vi "Auto Segement Extract.vi"(4 "Save Path":path, 5 "Sensor Data Array":dbl[][](array[numeric]), 7 "Title":string) -> (0 "End":dbl, 1 "Trimmed Segment":dbl[][](graph), 2 "No Peak Located":bool, 3 "Start":dbl)   [LabVIEW 2020]
uses:
  <vilib>/Utility/miscctls.llb/LVCursorListTypeDef.ctl
  <vilib>/Analysis/NI_AAL_SigProc.lvlib
panel:
  in  "OK Button":bool
  out "Last Sensor":dbl[](graph)
  out "First Sensor":dbl[](graph)
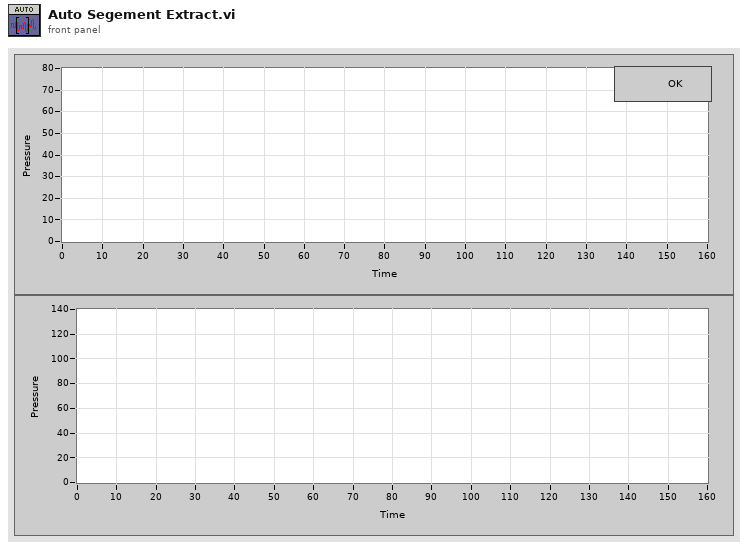
[diagram p1: front panel]
types:
  T1 = enum16{"open", "replace", "create", "open or create", "replace or create", "replace or create with confirmation"}
  T2 = typedef "LVCursorListTypeDef.ctl" = cluster{"Name":string, "Color":u32, "Style":u8, "Point Style":u8, "Name Visible":bool, "Allow Drag":bool, "Cursor Mode":u32, "Plot":i32, "Index":i32, "Position":cluster{"X":dbl, "Y":dbl}, "X Scale":u32, "Y Scale":u32, "Watch Plots":i32[], "Watch All Plots":bool, "Plot Area":i32, "Label Offset":cluster{"X":dbl, "Y":dbl}}[]
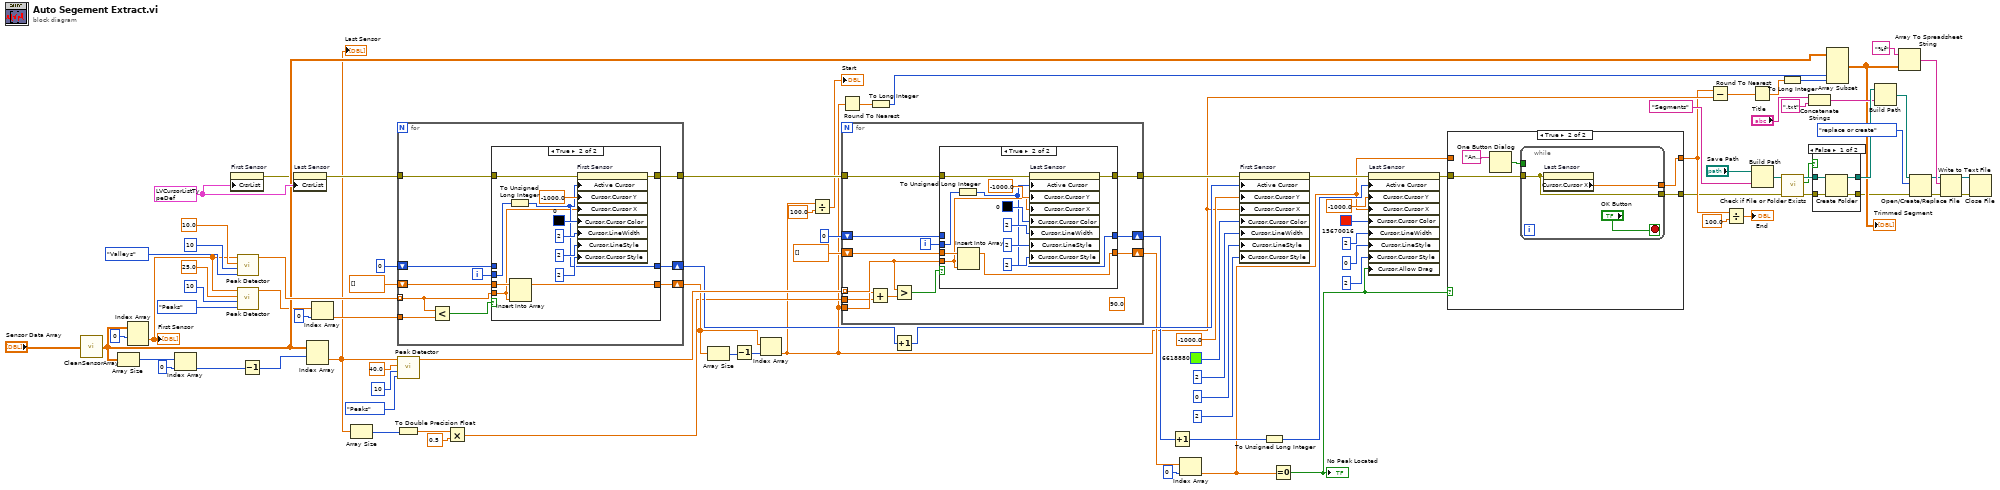
[diagram p0: block diagram]
diagram:
  w83 = T2 [{"Name"="", "Color"=0, "Style"=0, "Point Style"=0, "Name Visible"=FALSE, "Allow Drag"=FALSE, "Cursor Mode"=0, "Plot"=0, "Index"=0, "Position"={"X"=0.0, "Y"=0.0}, "X Scale"=0, "Y Scale"=0, "Watch Plots"=[], "Watch All Plots"=FALSE, "Plot Area"=0, "Label Offset"={"X"=0.0, "Y"=0.0}}, {"Name"="", "Color"=0, "Style"=0, "Point Style"=0, "Name Visible"=FALSE, "Allow Drag"=FALSE, "Cursor Mode"=0, "Plot"=0, "Index"=0, "Position"={"X"=0.0, "Y"=0.0}, "X Scale"=0, "Y Scale"=0, "Watch Plots"=[], "Watch All Plots"=FALSE, "Plot Area"=0, "Label Offset"={"X"=0.0, "Y"=0.0}}, {"Name"="", "Color"=0, "Style"=0, "Point Style"=0, "Name Visible"=FALSE, "Allow Drag"=FALSE, "Cursor Mode"=0, "Plot"=0, "Index"=0, "Position"={"X"=0.0, "Y"=0.0}, "X Scale"=0, "Y Scale"=0, "Watch Plots"=[], "Watch All Plots"=FALSE, "Plot Area"=0, "Label Offset"={"X"=0.0, "Y"=0.0}}, {"Name"="", "Color"=0, "Style"=0, "Point Style"=0, "Name Visible"=FALSE, "Allow Drag"=FALSE, "Cursor Mode"=0, "Plot"=0, "Index"=0, "Position"={"X"=0.0, "Y"=0.0}, "X Scale"=0, "Y Scale"=0, "Watch Plots"=[], "Watch All Plots"=FALSE, "Plot Area"=0, "Label Offset"={"X"=0.0, "Y"=0.0}}, {"Name"="", "Color"=0, "Style"=0, "Point Style"=0, "Name Visible"=FALSE, "Allow Drag"=FALSE, "Cursor Mode"=0, "Plot"=0, "Index"=0, "Position"={"X"=0.0, "Y"=0.0}, "X Scale"=0, "Y Scale"=0, "Watch Plots"=[], "Watch All Plots"=FALSE, "Plot Area"=0, "Label Offset"={"X"=0.0, "Y"=0.0}}, {"Name"="", "Color"=0, "Style"=0, "Point Style"=0, "Name Visible"=FALSE, "Allow Drag"=FALSE, "Cursor Mode"=0, "Plot"=0, "Index"=0, "Position"={"X"=0.0, "Y"=0.0}, "X Scale"=0, "Y Scale"=0, "Watch Plots"=[], "Watch All Plots"=FALSE, "Plot Area"=0, "Label Offset"={"X"=0.0, "Y"=0.0}}, {"Name"="", "Color"=0, "Style"=0, "Point Style"=0, "Name Visible"=FALSE, "Allow Drag"=FALSE, "Cursor Mode"=0, "Plot"=0, "Index"=0, "Position"={"X"=0.0, "Y"=0.0}, "X Scale"=0, "Y Scale"=0, "Watch Plots"=[], "Watch All Plots"=FALSE, "Plot Area"=0, "Label Offset"={"X"=0.0, "Y"=0.0}}, {"Name"="", "Color"=0, "Style"=0, "Point Style"=0, "Name Visible"=FALSE, "Allow Drag"=FALSE, "Cursor Mode"=0, "Plot"=0, "Index"=0, "Position"={"X"=0.0, "Y"=0.0}, "X Scale"=0, "Y Scale"=0, "Watch Plots"=[], "Watch All Plots"=FALSE, "Plot Area"=0, "Label Offset"={"X"=0.0, "Y"=0.0}}, {"Name"="", "Color"=0, "Style"=0, "Point Style"=0, "Name Visible"=FALSE, "Allow Drag"=FALSE, "Cursor Mode"=0, "Plot"=0, "Index"=0, "Position"={"X"=0.0, "Y"=0.0}, "X Scale"=0, "Y Scale"=0, "Watch Plots"=[], "Watch All Plots"=FALSE, "Plot Area"=0, "Label Offset"={"X"=0.0, "Y"=0.0}}, {"Name"="", "Color"=0, "Style"=0, "Point Style"=0, "Name Visible"=FALSE, "Allow Drag"=FALSE, "Cursor Mode"=0, "Plot"=0, "Index"=0, "Position"={"X"=0.0, "Y"=0.0}, "X Scale"=0, "Y Scale"=0, "Watch Plots"=[], "Watch All Plots"=FALSE, "Plot Area"=0, "Label Offset"={"X"=0.0, "Y"=0.0}}, {"Name"="", "Color"=0, "Style"=0, "Point Style"=0, "Name Visible"=FALSE, "Allow Drag"=FALSE, "Cursor Mode"=0, "Plot"=0, "Index"=0, "Position"={"X"=0.0, "Y"=0.0}, "X Scale"=0, "Y Scale"=0, "Watch Plots"=[], "Watch All Plots"=FALSE, "Plot Area"=0, "Label Offset"={"X"=0.0, "Y"=0.0}}, {"Name"="", "Color"=0, "Style"=0, "Point Style"=0, "Name Visible"=FALSE, "Allow Drag"=FALSE, "Cursor Mode"=0, "Plot"=0, "Index"=0, "Position"={"X"=0.0, "Y"=0.0}, "X Scale"=0, "Y Scale"=0, "Watch Plots"=[], "Watch All Plots"=FALSE, "Plot Area"=0, "Label Offset"={"X"=0.0, "Y"=0.0}}, {"Name"="", "Color"=0, "Style"=0, "Point Style"=0, "Name Visible"=FALSE, "Allow Drag"=FALSE, "Cursor Mode"=0, "Plot"=0, "Index"=0, "Position"={"X"=0.0, "Y"=0.0}, "X Scale"=0, "Y Scale"=0, "Watch Plots"=[], "Watch All Plots"=FALSE, "Plot Area"=0, "Label Offset"={"X"=0.0, "Y"=0.0}}, {"Name"="", "Color"=0, "Style"=0, "Point Style"=0, "Name Visible"=FALSE, "Allow Drag"=FALSE, "Cursor Mode"=0, "Plot"=0, "Index"=0, "Position"={"X"=0.0, "Y"=0.0}, "X Scale"=0, "Y Scale"=0, "Watch Plots"=[], "Watch All Plots"=FALSE, "Plot Area"=0, "Label Offset"={"X"=0.0, "Y"=0.0}}, {"Name"="", "Color"=0, "Style"=0, "Point Style"=0, "Name Visible"=FALSE, "Allow Drag"=FALSE, "Cursor Mode"=0, "Plot"=0, "Index"=0, "Position"={"X"=0.0, "Y"=0.0}, "X Scale"=0, "Y Scale"=0, "Watch Plots"=[], "Watch All Plots"=FALSE, "Plot Area"=0, "Label Offset"={"X"=0.0, "Y"=0.0}}, {"Name"="", "Color"=0, "Style"=0, "Point Style"=0, "Name Visible"=FALSE, "Allow Drag"=FALSE, "Cursor Mode"=0, "Plot"=0, "Index"=0, "Position"={"X"=0.0, "Y"=0.0}, "X Scale"=0, "Y Scale"=0, "Watch Plots"=[], "Watch All Plots"=FALSE, "Plot Area"=0, "Label Offset"={"X"=0.0, "Y"=0.0}}, {"Name"="", "Color"=0, "Style"=0, "Point Style"=0, "Name Visible"=FALSE, "Allow Drag"=FALSE, "Cursor Mode"=0, "Plot"=0, "Index"=0, "Position"={"X"=0.0, "Y"=0.0}, "X Scale"=0, "Y Scale"=0, "Watch Plots"=[], "Watch All Plots"=FALSE, "Plot Area"=0, "Label Offset"={"X"=0.0, "Y"=0.0}}, {"Name"="", "Color"=0, "Style"=0, "Point Style"=0, "Name Visible"=FALSE, "Allow Drag"=FALSE, "Cursor Mode"=0, "Plot"=0, "Index"=0, "Position"={"X"=0.0, "Y"=0.0}, "X Scale"=0, "Y Scale"=0, "Watch Plots"=[], "Watch All Plots"=FALSE, "Plot Area"=0, "Label Offset"={"X"=0.0, "Y"=0.0}}, {"Name"="", "Color"=0, "Style"=0, "Point Style"=0, "Name Visible"=FALSE, "Allow Drag"=FALSE, "Cursor Mode"=0, "Plot"=0, "Index"=0, "Position"={"X"=0.0, "Y"=0.0}, "X Scale"=0, "Y Scale"=0, "Watch Plots"=[], "Watch All Plots"=FALSE, "Plot Area"=0, "Label Offset"={"X"=0.0, "Y"=0.0}}, {"Name"="", "Color"=0, "Style"=0, "Point Style"=0, "Name Visible"=FALSE, "Allow Drag"=FALSE, "Cursor Mode"=0, "Plot"=0, "Index"=0, "Position"={"X"=0.0, "Y"=0.0}, "X Scale"=0, "Y Scale"=0, "Watch Plots"=[], "Watch All Plots"=FALSE, "Plot Area"=0, "Label Offset"={"X"=0.0, "Y"=0.0}}, {"Name"="", "Color"=0, "Style"=0, "Point Style"=0, "Name Visible"=FALSE, "Allow Drag"=FALSE, "Cursor Mode"=0, "Plot"=0, "Index"=0, "Position"={"X"=0.0, "Y"=0.0}, "X Scale"=0, "Y Scale"=0, "Watch Plots"=[], "Watch All Plots"=FALSE, "Plot Area"=0, "Label Offset"={"X"=0.0, "Y"=0.0}}, {"Name"="", "Color"=0, "Style"=0, "Point Style"=0, "Name Visible"=FALSE, "Allow Drag"=FALSE, "Cursor Mode"=0, "Plot"=0, "Index"=0, "Position"={"X"=0.0, "Y"=0.0}, "X Scale"=0, "Y Scale"=0, "Watch Plots"=[], "Watch All Plots"=FALSE, "Plot Area"=0, "Label Offset"={"X"=0.0, "Y"=0.0}}, {"Name"="Marker", "Color"=0, "Style"=0, "Point Style"=0, "Name Visible"=FALSE, "Allow Drag"=FALSE, "Cursor Mode"=0, "Plot"=0, "Index"=0, "Position"={"X"=0.0, "Y"=0.0}, "X Scale"=0, "Y Scale"=0, "Watch Plots"=[], "Watch All Plots"=FALSE, "Plot Area"=0, "Label Offset"={"X"=0.0, "Y"=0.0}}] ("Cursor List")
  n1 = call "CleanSensorArray.vi"("Sensor Data Array"="Sensor Data Array") -> ("Clean Array"=w77:dbl[][])  [unwired: 4 in]
  n2 = Array Size(array=w77) -> (size(s)=w90:i32[])
  n3 = Index Array(array=w77, index (row)=0) -> (element=w44:dbl[])  [unwired: 1 in]
  "First Sensor" <- w44
  n4 = Index Array(array=w90, index=0) -> (element=w88:i32)
  n5 = property on="First Sensor" class="WFGraph (strict)"("CrsrList"=w83) -> (error out=w59:errorcluster)  [unwired: 2 in, 1 out]
  n6 = call <vilib>:"Peak Detector.vi"("peaks/valleys"=enum32{"Peaks", "Valleys"}."Valleys", "width"=10, "threshold"=10.0, "X"=w44) -> ("Locations"=w85:dbl[])  [unwired: 3 in, 4 out]
  n7 = call <vilib>:"Peak Detector.vi"("peaks/valleys"=enum32{"Peaks", "Valleys"}."Peaks", "width"=10, "threshold"=25.0, "X"=w44) -> ("Locations"=w53:dbl[])  [unwired: 3 in, 4 out]
  n8 = Decrement(x=w88) -> (x-1=w87:i32)
  n9 = property on="Last Sensor" class="WFGraph (strict)"(error in=w59, "CrsrList"=w83) -> (error out=w58:errorcluster)  [unwired: 1 in, 1 out]
  n10 = Index Array(array=w77, index (row)=w87) -> (element=w42:dbl[])  [unwired: 1 in]
  "Last Sensor" <- w42
  n11 = Index Array(array=w53, index=0) -> (element=w51:dbl)
  n12 = Array Size(array=w42) -> (size(s)=w41:i32)
  n13 = for {
    tunnel: w85 -> [w99] mode=indexing
    tunnel: w58 -> [w101]
    tunnel: [w100] -> w57
    tunnel: w51 -> [w98]
    shift-right: [w95] -> w47
    shift-left: dbl[] [] -> [w96]
    shift-right: [w93] -> w48
    shift-left: u32 0 -> [w94]
    i -> [w102]
    n14 = Less?(x=w99, y=w98) -> (x < y?=w97:bool)
    n15 = case shown="True" w97 {
      tunnel: w102 -> [_ w114]
      tunnel: w99 -> [_ w106]
      tunnel: [w103 w111] -> w93
      tunnel: w101 -> [w105 w110]
      tunnel: [w105 w109] -> w100
      tunnel: w96 -> [w104 w108]
      tunnel: [w104 w107] -> w95
      tunnel: w94 -> [w103 _]
      frame False {
      }
      frame True {
        n16 = To Unsigned Long Integer(number=w114) -> (unsigned 32bit integer=w111:u32)
        n17 = Insert Into Array(array=w108, new element=w106) -> (w107:dbl[])  [unwired: 1 in]
        n18 = property on="First Sensor" class="WFGraph (strict)"(error in=w110, "Active Cursor"=w111, "Cursor.Cursor Y"=-1000.0 ("Cursor.Cursor Position:Cursor Y"), "Cursor.Cursor X"=w106, "Cursor.Cursor Color"=u32 0, "Cursor.LineWidth"=u8 2 ("Cursor.Line Width"), "Cursor.LineStyle"=u8 2 ("Cursor.Line Style"), "Cursor.Cursor Style"=u8 2) -> (error out=w109:errorcluster)  [unwired: 1 in, 1 out]
      }
    }
  }
  n19 = call <vilib>:"Peak Detector.vi"("peaks/valleys"=enum32{"Peaks", "Valleys"}."Peaks", "width"=10, "threshold"=40.0, "X"=w42) -> ("Locations"=w84:dbl[])  [unwired: 3 in, 4 out]
  n20 = To Double Precision Float(number=w41) -> (double precision float=w40:dbl)
  n21 = Multiply(x=w40, y=0.5) -> (x*y=w38:dbl)
  n22 = Array Size(array=w47) -> (size(s)=w46:i32)
  n23 = Decrement(x=w46) -> (x-1=w45:i32)
  n24 = Index Array(array=w47, index=w45) -> (element=w35:dbl)
  n25 = Divide(x=w35, y=100.0) -> (x/y=→"Start":dbl)
  n26 = Round To Nearest(number=w35) -> (nearest integer value=w73:dbl)
  n27 = for {
    tunnel: w84 -> [w127] mode=indexing
    tunnel: w57 -> [w120]
    tunnel: w35 -> [w126]
    shift-right: [w123] -> w63
    shift-left: dbl[] [] -> [w124]
    shift-right: [w121] -> w61
    shift-left: u32 0 -> [w122]
    tunnel: [w119] -> w60
    tunnel: w38 -> [w118]
    i -> [w129]
    (unwired) 90.0 ("y")
    n28 = Add(x=w126, y=w118) -> (x+y=w125:dbl)
    n29 = Greater?(x=w127, y=w125) -> (0:w128:bool)
    n30 = case shown="True" w128 {
      tunnel: w129 -> [_ w141]
      tunnel: w127 -> [_ w136]
      tunnel: w124 -> [w132 w138]
      tunnel: [w132 w137] -> w123
      tunnel: w122 -> [w131 _]
      tunnel: [w131 w135] -> w121
      tunnel: w120 -> [w130 w134]
      tunnel: [w130 w133] -> w119
      frame False {
      }
      frame True {
        n31 = To Unsigned Long Integer(number=w141) -> (unsigned 32bit integer=w135:u32)
        n32 = Insert Into Array(array=w138, new element=w136) -> (w137:dbl[])  [unwired: 1 in]
        n33 = property on="Last Sensor" class="WFGraph (strict)"(error in=w134, "Active Cursor"=w135, "Cursor.Cursor Y"=-1000.0 ("Cursor.Cursor Position:Cursor Y"), "Cursor.Cursor X"=w136, "Cursor.Cursor Color"=u32 0, "Cursor.LineWidth"=u8 2 ("Cursor.Line Width"), "Cursor.LineStyle"=u8 2 ("Cursor.Line Style"), "Cursor.Cursor Style"=u8 2) -> (error out=w133:errorcluster)  [unwired: 1 in, 1 out]
      }
    }
  }
  n34 = To Long Integer(number=w73) -> (32bit integer=w75:i32)
  n35 = Increment(x=w48) -> (x+1=w65:u32)
  n36 = Increment(x=w61) -> (x+1=w64:u32)
  n37 = Index Array(array=w63, index=0) -> (element=w3:dbl)
  n38 = property on="First Sensor" class="WFGraph (strict)"(error in=w60, "Active Cursor"=w65, "Cursor.Cursor Y"=-1000.0 ("Cursor.Cursor Position:Cursor Y"), "Cursor.Cursor X"=w35, "Cursor.Cursor Color"=u32 6618880, "Cursor.LineWidth"=u8 2 ("Cursor.Line Width"), "Cursor.LineStyle"=u8 0 ("Cursor.Line Style"), "Cursor.Cursor Style"=u8 2) -> (error out=w12:errorcluster)  [unwired: 1 in, 1 out]
  n39 = To Unsigned Long Integer(number=w64) -> (unsigned 32bit integer=w11:u32)
  n40 = Equal To 0?(x=w3) -> (x = 0?=w4:bool)
  "No Peak Located" <- w4
  n41 = property on="Last Sensor" class="WFGraph (strict)"(error in=w12, "Active Cursor"=w11, "Cursor.Cursor Y"=-1000.0 ("Cursor.Cursor Position:Cursor Y"), "Cursor.Cursor X"=w3, "Cursor.Cursor Color"=u32 15670016, "Cursor.LineWidth"=u8 2 ("Cursor.Line Width"), "Cursor.LineStyle"=u8 0 ("Cursor.Line Style"), "Cursor.Cursor Style"=u8 2, "Cursor.Allow Drag"=w4) -> (error out=w2:errorcluster)  [unwired: 1 in, 1 out]
  n42 = case shown="True" w4 {
    tunnel: [w146 w151] -> w5
    tunnel: w3 -> [w146 _]
    tunnel: w2 -> [w145 w148]
    tunnel: [w145 w147] -> w1
    frame False {
    }
    frame True {
      n43 = One Button Dialog(message="An end-swallow peak could not be located. Please mark it manually.") -> (true=w149:bool)  [unwired: 1 in]
      n44 = while {
        tunnel: [w154] -> w151
        tunnel: w149 -> [_]
        tunnel: w148 -> [w152]
        tunnel: [w152] -> w147
        stop <- "OK Button" stop-if-true
        n45 = property on="Last Sensor" class="WFGraph (strict)"(error in=w152) -> ("Cursor.Cursor X"=w154:dbl)  [unwired: 1 in, 2 out]
      }
    }
  }
  n46 = Subtract(x=w5, y=w35) -> (x-y=w72:dbl)
  n47 = Divide(x=w5, y=100.0) -> (x/y=→"End":dbl)
  n48 = Round To Nearest(number=w72) -> (nearest integer value=w71:dbl)
  n49 = Build Path(base path="Save Path", name or relative path="Segments") -> (appended path=w29:path)
  n50 = To Long Integer(number=w71) -> (32bit integer=w74:i32)
  n51 = call <vilib>:"Check if File or Folder Exists.vi"("error in (no error)"=w1, "path"=w29) -> ("error out"=w27:errorcluster, "file or folder exists?"=w26:bool, "dup path"=w28:path)  [unwired: 7 in]
  n52 = Concatenate Strings("Title", ".txt" ("string")) -> (w23:string)
  n53 = case shown="False" w26 {
    tunnel: w28 -> [w158 w160]
    tunnel: w27 -> [w157 w159]
    tunnel: [w156 w159] -> w13
    tunnel: [w155 w160] -> w25
    frame False {
      n54 = Create Folder(path (use dialog)=w158, error in=w157) -> (created path=w155:path, error out=w156:errorcluster)  [unwired: 1 in, 1 out]
    }
    frame True {
    }
  }
  n55 = Array Subset(array=w77, index (col)=w75, length (col)=w74) -> (w21:dbl[][])  [unwired: 2 in]
  "Trimmed Segment" <- w21
  n56 = Build Path(base path=w25, name or relative path=w23) -> (appended path=w14:path)
  n57 = Array To Spreadsheet String(array=w21, 3:"%f" ("format string")) -> (spreadsheet string=w24:string)  [unwired: 1 in]
  n58 = Open/Create/Replace File(file path (use dialog)=w14, error in=w13, operation (0:open)=T1."replace or create") -> (refnum out=w18:refnum<file>, error out=w19:errorcluster)  [unwired: 3 in, 1 out]
  n59 = Write to Text File(file (use dialog)=w18, text=w24, error in=w19) -> (refnum out=w16:refnum<file>, error out=w17:errorcluster)  [unwired: 1 in, 1 out]
  n60 = Close File(refnum=w16, error in=w17) -> ()  [unwired: 2 out]
